vi "Get SR Number List.vi"(4 "list in":T1[](array[typedef]) {"Creation Date" format="%<%x>T"; "Last Updated" format="%<%x>T"}) -> (1 "SR number array out":i32[](array[numeric]))   [LabVIEW 2018]
uses:
  SR Cluster.ctl
  SR Status.ctl
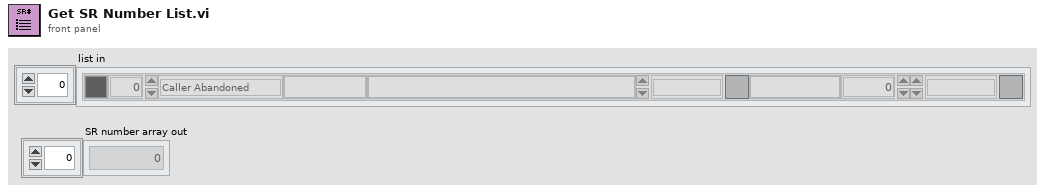
[diagram p1: front panel]
types:
  T1 = typedef "SR Cluster.ctl" = cluster{"Color":u32, "SR Number":i32, "SR Status":T2, "SR Type":string, "Summary":string, "Last Updated":timestamp, "Service Level":string, "Days Open":dbl, "Creation Date":timestamp}
  T2 = typedef "SR Status.ctl" = enum16{"Caller Abandoned", "Created in Error", "Expired", "Forum Resolved AE", "Forum Resolved Customer", "IN WORK", "IN WORK Collab with AES", "IN WORK Collab with PSE", "IN WORK Collab with SE", "IN WORK Customer Added Note", "IN WORK Escalation", "IN WORK Wait on Customer", "Open", "Potentially Resolved", "Presumed Resolved", "RMA Approved for Return", "Resolved", "Passed Off"}
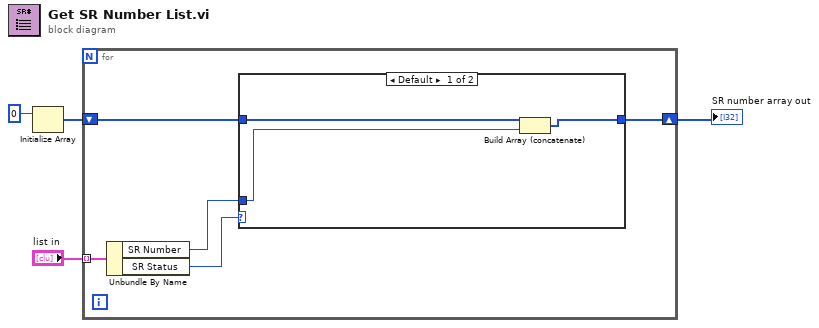
[diagram p0: block diagram]
diagram:
  n1 = Initialize Array(0 ("SR Number")) -> (w2:i32[])  [unwired: 1 in]
  n2 = for {
    tunnel: "list in" -> [w9] mode=indexing
    shift-right: [w7] -> w1
    shift-left: w2 -> [w8]
    n3 = Unbundle By Name(w9) -> ("SR Number"=w6:i32, "SR Status"=w5:T2)
    n4 = case shown="Default" w5 {
      tunnel: w8 -> [w12 w13]
      tunnel: [w11 w13] -> w7
      tunnel: w6 -> [w10 _]
      frame Default {
        n5 = Build Array (concatenate)(w12, w10) -> (w11:i32[])
      }
      frame "Created in Error", "Presumed Resolved".."Resolved" {
      }
    }
  }
  "SR number array out" <- w1
